vi "Clear Scan Time Out_2_test2.vi"(6 "Channel number":i32, 7 "ESP32 ref":refnum<visa-resource-name>="COM4", 8 "error in (no error)":errorcluster, 11 "VISA Refnum in":refnum<visa-resource-name>) -> (0 "error out":errorcluster, 1 "error?":bool, 2 "Time out count":i32, 3 "VISA Refnum out":refnum<visa-resource-name>, 5 "ESP32 ref out":refnum<visa-resource-name>)   [LabVIEW 2023]
uses:
  <vilib>/Utility/error.llb/DialogType.ctl
  <instrlib>/Agilent 3446X Series/Agilent 3446X Series.lvlib
panel:
  in  "Boolean":bool
  in  "milliseconds to wait":u32
  out "Measurements":dbl[](array[numeric])
  out "x != y?":bool
  out "error out 3":errorcluster
  out "error out 2":errorcluster
  out "Measurements 3":dbl[](array[numeric])
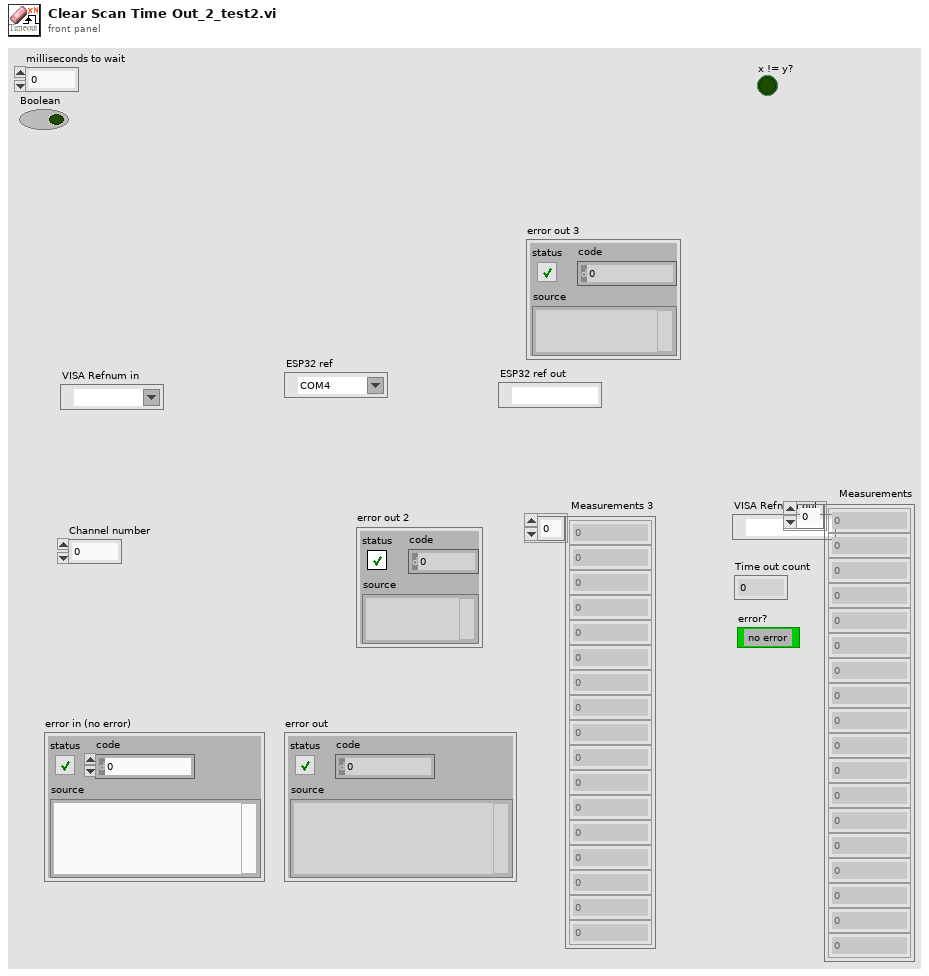
[diagram p1: front panel]
types:
  T1 = typedef "DialogType.ctl" = u16
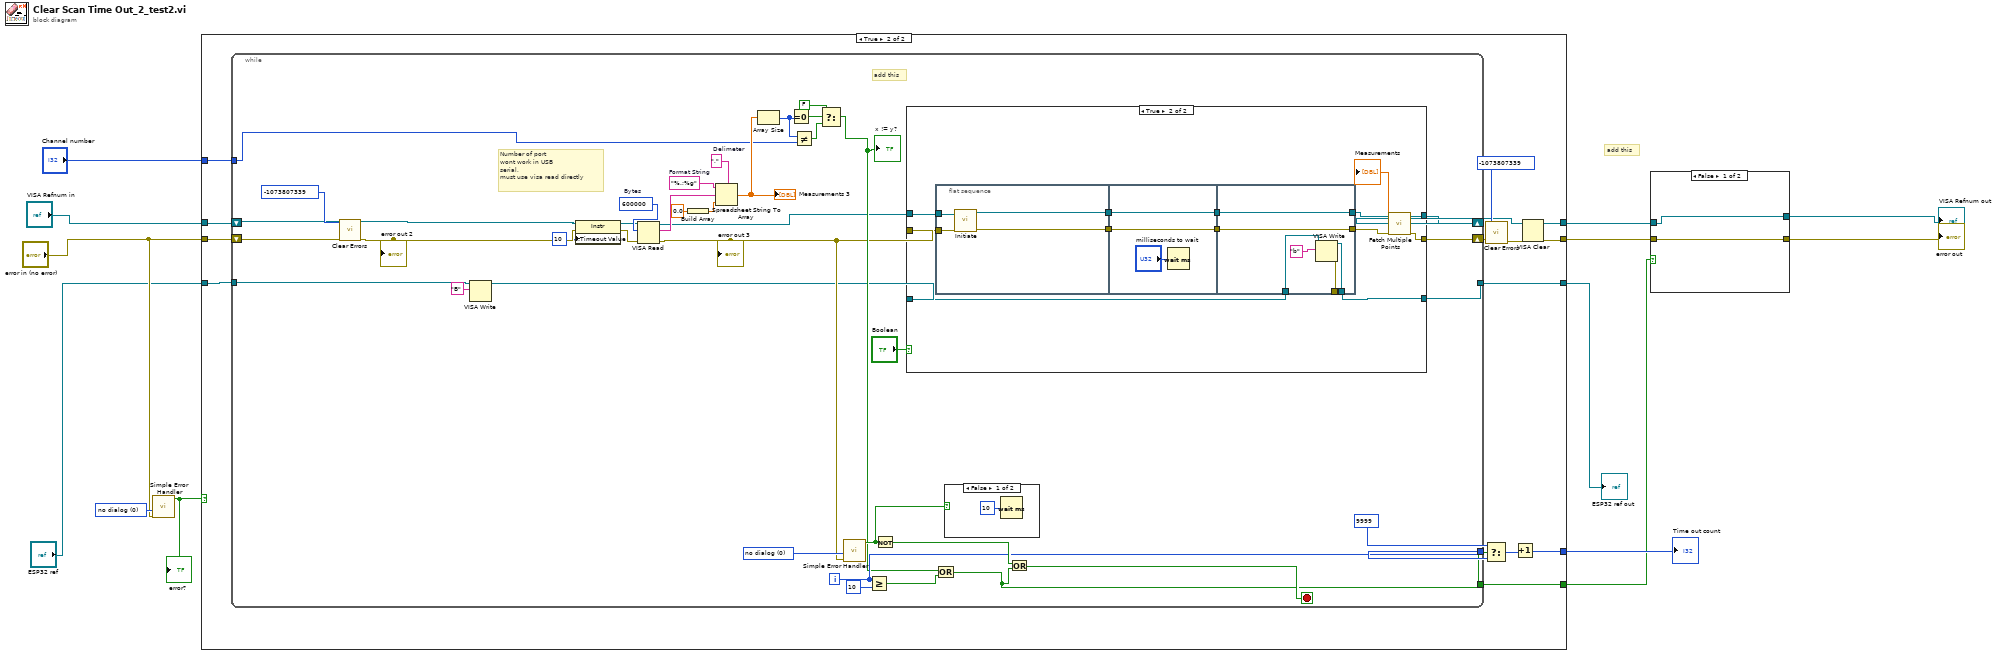
[diagram p0: block diagram]
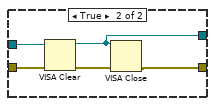
[diagram p2: hidden frame]
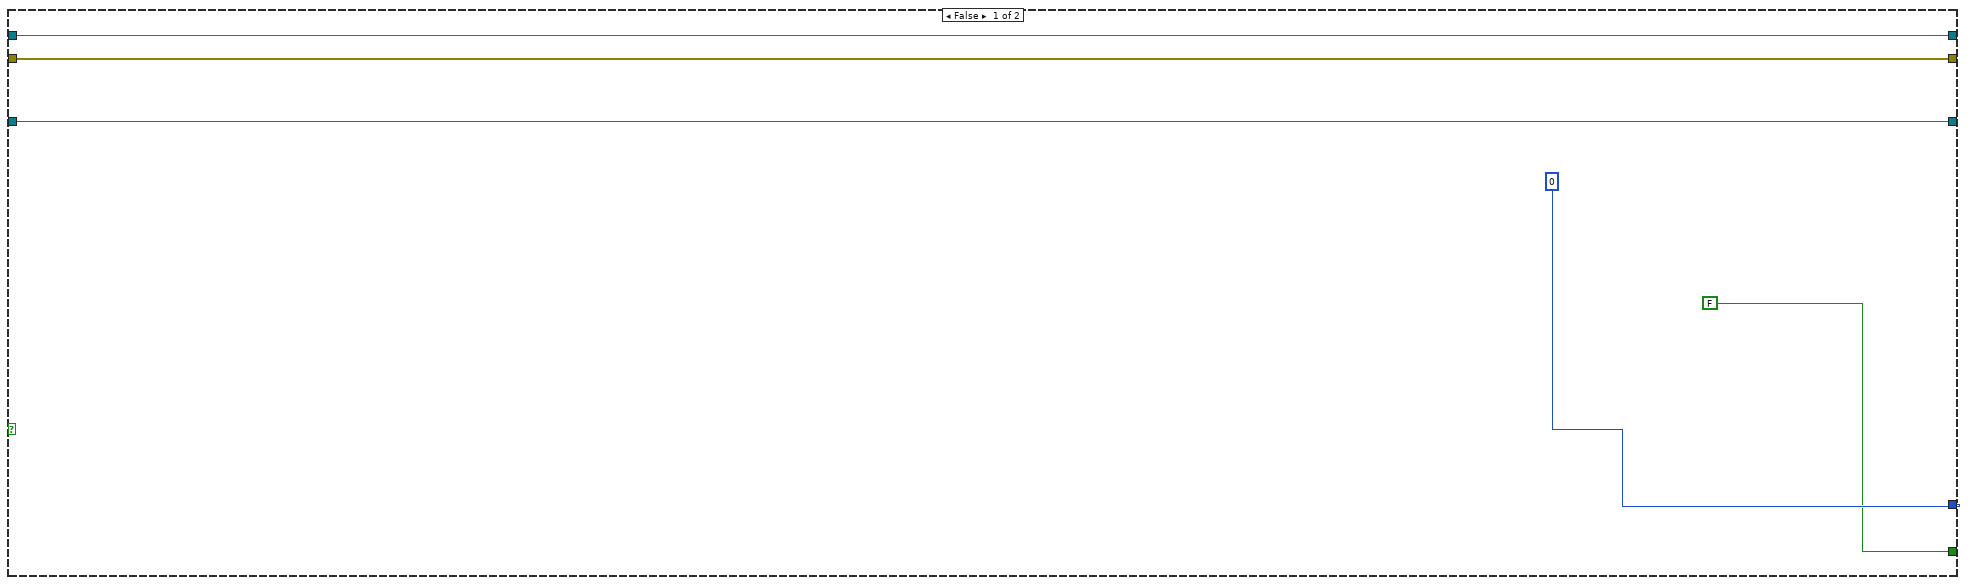
[diagram p3: hidden frame]
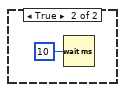
[diagram p5: hidden frame]
diagram:
  w12 = T1 0 items=["no dialog", "OK message", "continue or stop message", "OK message + warnings", "continue/stop + warnings"] ("type of dialog (OK msg:1)")
  # "add this"
  n1 = call <vilib>:"Simple Error Handler.vi"("type of dialog (OK msg:1)"=w12, "error in (no error)"="error in (no error)") -> ("error?"=w10:bool)  [unwired: 3 in, 4 out]
  "error?" <- w10
  n2 = case shown="True" w10 {
    tunnel: [w18 w19] -> w4
    tunnel: "error in (no error)" -> [w17 w34]
    tunnel: "VISA Refnum in" -> [w18 w33]
    tunnel: [w17 w21] -> w3
    tunnel: [0 w32] -> w9
    tunnel: "ESP32 ref" -> [w15 w28]
    tunnel: [w15 w27] -> w7
    tunnel: "Channel number" -> [_ w26]
    tunnel: [FALSE w23] -> w5
    frame False {
    }
    frame True {
      n3 = while {
        shift-right: [w38] -> w25
        shift-left: w34 -> [w70]
        shift-right: [w39] -> w20
        shift-left: w33 -> [w52]
        tunnel: [w64] -> w30
        tunnel: [w47] -> w23
        tunnel: w28 -> [w51]
        tunnel: [w36] -> w27
        tunnel: w26 -> [w49]
        i -> [w64]
        stop <- w65 stop-if-true
        w60 = ","  # Delimeter
        w61 = "%.;%g"  # Format String
        w56 = u32 600000  # Bytes
        w68 = T1 0 items=["no dialog", "OK message", "continue or stop message", "OK message + warnings", "continue/stop + warnings"] ("type of dialog (OK msg:1)")
        # "add this"
        # "Number of port\nwont work in USB \nserial,\nmust use visa read directly"
        n4 = call <vilib>:"Clear Errors.vi"("error in (no error)"=w70, "specific error code to clear (0: all)"=-1073807339 ("code out")) -> ("error out"=w69:errorcluster)  [unwired: 4 in, 1 out]
        "error out 2" <- w69
        n5 = VISA Write(VISA resource name=w51, write buffer="B") -> (VISA resource name out=w37:refnum<visa-resource-name>)  [unwired: 1 in, 2 out]
        n6 = property class="Instr"(reference=w52, error in=w69, "General Settings:Timeout Value"=u32 10) -> (reference out=w55:refnum<visa-resource-name>, error out=w54:errorcluster)
        n7 = VISA Read(VISA resource name=w55, byte count=w56, error in (no error)=w54) -> (VISA resource name out=w41:refnum<visa-resource-name>, read buffer=w57:string, error out=w40:errorcluster)  [unwired: 1 out]
        "error out 3" <- w40
        n8 = Build Array(0.0) -> (w58:dbl[])
        n9 = Spreadsheet String To Array(delimiter (Tab)=w60, format string=w61, spreadsheet string=w57, array type (2D Dbl)=w58) -> (array=w50:dbl[])
        "Measurements 3" <- w50
        n10 = Array Size(array=w50) -> (size(s)=w42:i32)
        n11 = Equal To 0?(x=w42) -> (x = 0?=w46:bool)
        n12 = Not Equal?(x=w42, y=w49) -> (x != y?=w45:bool)
        n13 = Select(t=FALSE, s=w46, f=w45) -> (s? t:f=w43:bool)
        "x != y?" <- w43
        n14 = call <vilib>:"Simple Error Handler.vi"("type of dialog (OK msg:1)"=w68, "error in (no error)"=w40) -> ("error?"=w63:bool)  [unwired: 3 in, 4 out]
        n15 = Greater Or Equal?(x=w64, y=10) -> (x >= y?=w48:bool)
        n16 = Not(x=w63) -> (.not. x?=w66:bool)
        n17 = case shown="True" "Boolean" {
          tunnel: w41 -> [w74 w83]
          tunnel: w40 -> [w73 w82]
          tunnel: [w74 w79] -> w39
          tunnel: [w73 w78] -> w38
          tunnel: w37 -> [w72 w77]
          tunnel: [w72 w76] -> w36
          frame False {
          }
          frame True {
            n18 = flat-sequence {
              tunnel: [w91] -> w87
              tunnel: [w90] -> w86
              tunnel: w83 -> [w89]
              tunnel: w82 -> [w88]
              tunnel: w87 -> [w94]
              tunnel: [w94] -> w85
              tunnel: w86 -> [w93]
              tunnel: [w93] -> w84
              tunnel: w85 -> [w100]
              tunnel: w84 -> [w99]
              tunnel: w77 -> [w98]
              tunnel: [w97] -> w76
              tunnel: [w96] -> _
              tunnel: [w100] -> w80
              tunnel: [w99] -> w81
              frame #0 {
                n19 = call <instrlib>:"Initiate.vi"("error in (no error)"=w88, "VISA resource name"=w89) -> ("error out"=w91:errorcluster, "VISA resource name out"=w90:refnum<visa-resource-name>)  [unwired: 8 in]
              }
              frame #1 {
                n20 = Wait (ms)(milliseconds to wait="milliseconds to wait") -> ()  [unwired: 1 out]
              }
              frame #2 {
                n21 = VISA Write(VISA resource name=w98, write buffer="b" ("data in")) -> (VISA resource name out=w97:refnum<visa-resource-name>, error out=w96:errorcluster)  [unwired: 1 in, 1 out]
              }
            }
            n22 = call <instrlib>:"Fetch Multiple Points.vi"("error in (no error)"=w80, "VISA resource name"=w81) -> ("error out"=w78:errorcluster, "Measurements"=→"Measurements":dbl[], "VISA resource name out"=w79:refnum<visa-resource-name>)  [unwired: 2 in, 5 out]
          }
        }
        n23 = Or(x=w43, y=w48) -> (x .or. y?=w47:bool)
        n24 = case shown="False" w63 {
          frame False {
            n25 = Wait (ms)(milliseconds to wait=u32 10) -> ()  [unwired: 1 out]
          }
          frame True {
            n26 = Wait (ms)(milliseconds to wait=u32 10) -> ()  [unwired: 1 out]
          }
        }
        n27 = Or(x=w66, y=w47) -> (x .or. y?=w65:bool)
      }
      n28 = Select(t=9999, s=w23, f=w30) -> (s? t:f=w31:i32)
      n29 = call <vilib>:"Clear Errors.vi"("error in (no error)"=w25, "specific error code to clear (0: all)"=-1073807339 ("code out")) -> ("error out"=w22:errorcluster)  [unwired: 4 in, 1 out]
      n30 = Increment(x=w31) -> (x+1=w32:i32)
      n31 = VISA Clear(VISA resource name=w20, error in (no error)=w22) -> (VISA resource name out=w19:refnum<visa-resource-name>, error out=w21:errorcluster)
    }
  }
  "Time out count" <- w9
  "ESP32 ref out" <- w7
  n32 = case shown="False" w5 {
    tunnel: w4 -> [w104 w108]
    tunnel: w3 -> [w103 w109]
    tunnel: [w103 w106] -> w2
    tunnel: [w104 w105] -> w1
    frame False {
    }
    frame True {
      n33 = VISA Clear(VISA resource name=w108, error in (no error)=w109) -> (VISA resource name out=w105:refnum<visa-resource-name>, error out=w107:errorcluster)
      n34 = VISA Close(VISA resource name=w105, error in (no error)=w107) -> (error out=w106:errorcluster)
    }
  }
  "error out" <- w2
  "VISA Refnum out" <- w1
